vi "GenerateTriggeredStimulus.vi"(8 "error in (no error)":errorcluster, 11 "Stimulus in":refnum<class "StimulusObject.lvclass">) -> (0 "error out":errorcluster, 2 "TriggeredStimulus":sgl[][](array[numeric]), 3 "Stimulus out":refnum<class "StimulusObject.lvclass">)   [LabVIEW 2019, in "StimulusObject.lvclass"]
uses:
  StimulusObject.lvclass
  ParametersGlobal.vi
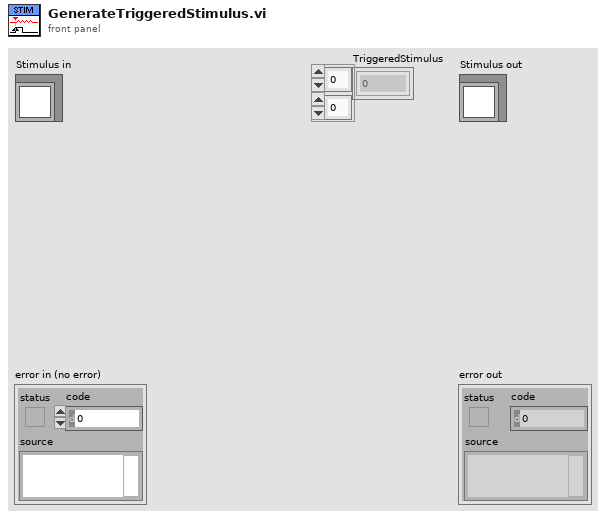
[diagram p1: front panel]
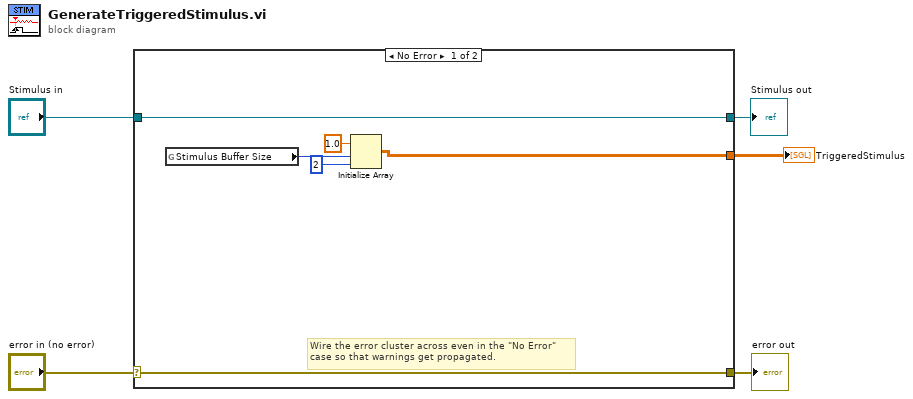
[diagram p0: block diagram]
diagram:
  n1 = case shown="No Error" "error in (no error)" {
    selector: "error in (no error)" -> [w11 w13]
    tunnel: [w11 w13] -> w4
    tunnel: [w8 w12] -> w2
    tunnel: "Stimulus in" -> [w8 w12]
    tunnel: [w6 _] -> w1
    frame No Error {
      # "Wire the error cluster across even in the \"No Error\"\ncase so that warnings get propagated."
      n2 = global read "ParametersGlobal.vi" "Stimulus Buffer Size"() -> (w7:i32)
      n3 = Initialize Array(sgl 1.0 ("element"), w7, 2 ("dimension size")) -> (w6:sgl[][])
    }
    frame Error {
    }
  }
  "error out" <- w4
  "Stimulus out" <- w2
  "TriggeredStimulus" <- w1
